vi "Start.vi"(8 "error in (no error)":errorcluster, 10 "Message in":refnum<class "StartMessage.lvclass">, 11 "Galvo in":refnum<class "InVivo_ImagingModeSPIM.lvclass">) -> (0 "error out":errorcluster, 3 "Galvo out":refnum<class "InVivo_ImagingModeSPIM.lvclass">)   [LabVIEW 2012, in "InVivo_ImagingModeSPIM.lvclass"]
doc: "This member function is called when the statemachine in the run.vi receives an 'start' command. It relays the message to all observers of the component.\n\nOverride this member function in your derived class if you need additional start functionality (but don't forget to call the parent method)."
uses:
  InVivo_ImagingModeSPIM.lvclass
  <vilib>/Distrio/Murmex/StartMessage/StartMessage.lvclass
  <vilib>/Distrio/Murmex/Murmex/Murmex.lvclass
  <vilib>/Distrio/Murmex/StartMessage/run mode enum.ctl
  <vilib>/Distrio/Murmex/ProceedMessage/ProceedMessage.lvclass
  InVivo_ImagingModeSPIM.lvclass/InVivo_ImagingModeSPIM.ctl
  <vilib>/Distrio/Murmex/StartMessage/Get run mode.vi
panel:
  # "This member function is called when the statemachine in the run.vi receives an 'start' command. It relays the message to all observers of the component.\n\nOverride this member function in your derived class if you need additional start functionality (but don't forget to call the parent method)."
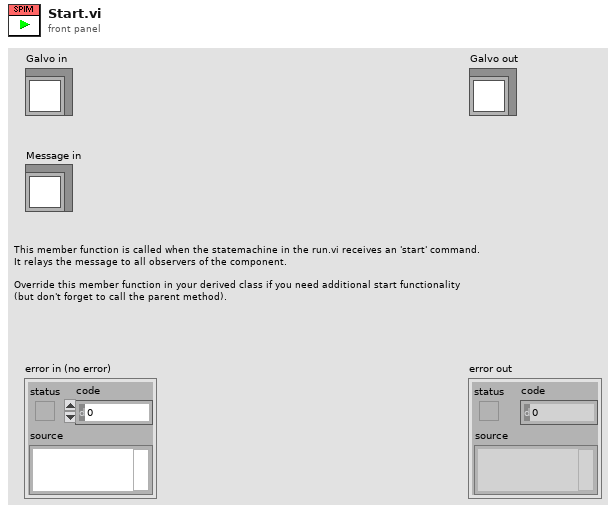
[diagram p1: front panel]
types:
  T1 = typedef "Murmex.lvlib/StartMessage.lvclass/run mode enum.ctl" = enum16{"infinite", "finite"}
  T2 = enum8{"Enabled", "Disabled", "Disabled and Grayed Out"}
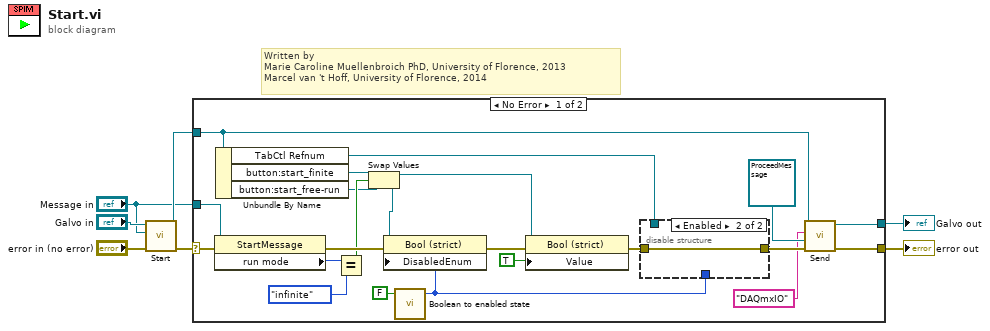
[diagram p0: block diagram]
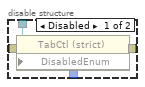
[diagram p2: hidden frame]
diagram:
  # "Written by \nMarie Caroline Muellenbroich PhD, University of Florence, 2013 \nMarcel van 't Hoff, University of Florence, 2014"
  n1 = call-parent "Start.vi"("error in (no error)"="error in (no error)", "Message in"="Message in", "Murmex in"="Galvo in") -> ("error out"=w4:errorcluster, "Murmex out"=w5:refnum<class "InVivo_ImagingModeSPIM.lvclass">)  [unwired: 7 in]
  n2 = case shown="No Error" w4 {
    selector: w4 -> [w26 w36]
    tunnel: w5 -> [w25 w35]
    tunnel: [w29 w36] -> w3
    tunnel: [w28 w35] -> w2
    tunnel: "Message in" -> [w27 _]
    frame No Error {
      n3 = property class="StartMessage"(reference=w27, error in=w26) -> (error out=w21:errorcluster, "run mode"=w24:T1)  [unwired: 1 out]
      n4 = Unbundle By Name(w25) -> ("TabCtl Refnum"=w20:refnum<vi>, "button:start_finite"=w16:refnum<vi>, "button:start_free-run"=w15:refnum<vi>)
      n5 = Equal?(x=w24, y=run_mode_enum."infinite" ("run mode")) -> (x = y?=w17:bool)
      n6 = Swap Values(12:w16, 13:w17, 14:w15) -> (1:w11:refnum<vi>, 3:w10:refnum<vi>)
      n7 = call <vilib>:"Boolean to enabled state.vi"("boolean in"=FALSE) -> ("enabled status out"=w19:T2)  [unwired: 4 in]
      n8 = property class="Bool (strict)"(reference=w10, error in=w21, "DisabledEnum"=w19) -> (error out=w13:errorcluster)  [unwired: 1 out]
      n9 = property class="Bool (strict)"(reference=w11, error in=w13, "Value"=TRUE) -> (error out=w12:errorcluster)  [unwired: 1 out]
      n10 = disable-structure shown="Enabled" {
        disable-tunnel: w20 -> [w33 _]
        disable-tunnel: w19 -> [w32 _]
        disable-tunnel: [w31 w34] -> w18
        disable-tunnel: w12 -> [w30 w34]
        frame Disabled {
          n11 = property class="TabCtl (strict)"(reference=w33, error in=w30, "DisabledEnum"=w32) -> (error out=w31:errorcluster)  [unwired: 1 out]
        }
        frame Enabled {
        }
      }
      n12 = call <vilib>:"Send.vi"("error in (no error)"=w18, "Message"=refnum<class "ProceedMessage.lvclass"> refnum ("Murmex.lvlib:ProceedMessage"), "recipient"="DAQmxIO", "Murmex in"=w25) -> ("error out"=w29:errorcluster, "Murmex out"=w28:refnum<class "InVivo_ImagingModeSPIM.lvclass">)  [unwired: 6 in]
    }
    frame Error {
    }
  }
  "error out" <- w3
  "Galvo out" <- w2
